vi "Check Action.vi"(6 "HRS Time":dbl, 7 "Values In":dbl[](array[numeric]), 8 "error in (no error)":errorcluster, 11 "Valve in":refnum<class "PeriodicControl.lvclass">) -> (0 "error out":errorcluster, 1 "Do Action":bool, 2 "Action":T1, 3 "Valve out":refnum<class "PeriodicControl.lvclass">, 5 "Values":dbl[](array[numeric]))   [LabVIEW 2020, in "VolatusControl.lvlib" / "PeriodicControl.lvclass"]
uses:
  PeriodicControl.lvclass
  Valve Action.ctl
  Volatus/MessageQ/MessageQ.lvclass
  PeriodicControl.lvclass/PeriodicControl.ctl
  State.ctl
  VolatusControl.lvlib
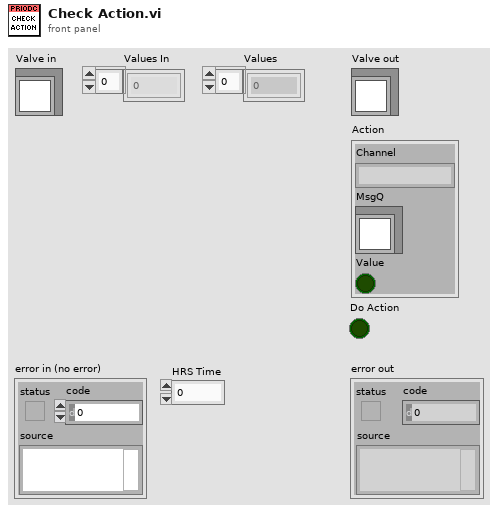
[diagram p1: front panel]
types:
  T1 = typedef "VolatusControl.lvlib/Valve Action.ctl" = cluster{"Channel":string, "MsgQ":refnum<class "MessageQ.lvclass">, "Value":bool}
  T2 = typedef "VolatusControl.lvlib/PeriodicControl.lvclass/State.ctl" = enum16{"Idle", "Start", "Run", "Stop"}
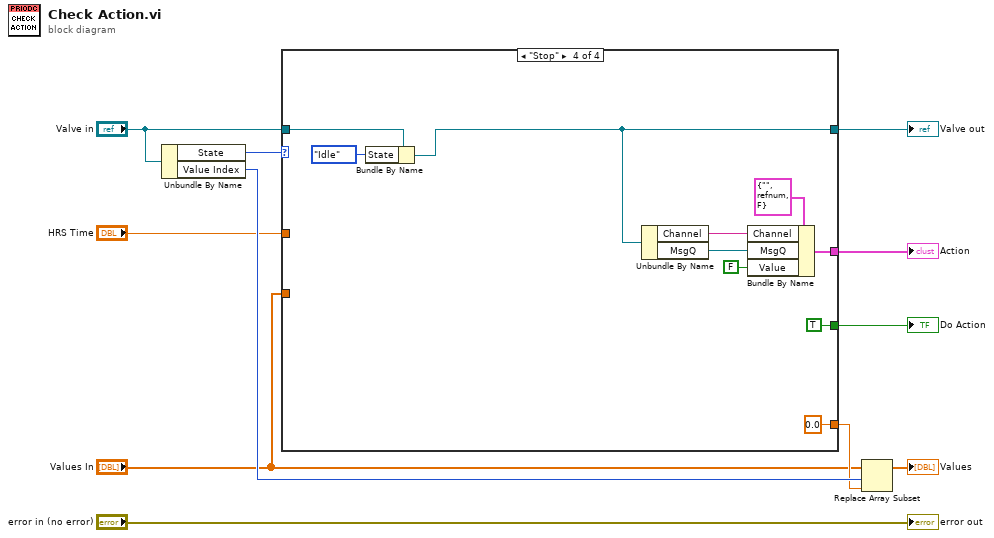
[diagram p0: block diagram]
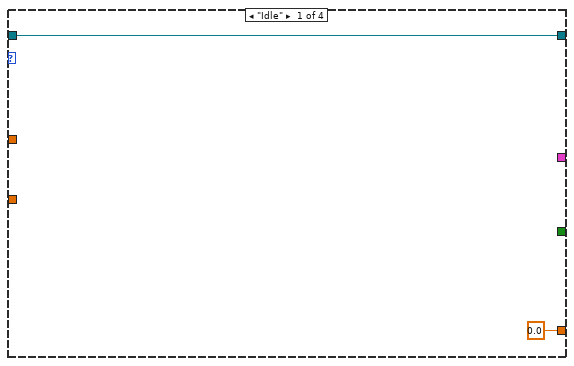
[diagram p2: hidden frame]
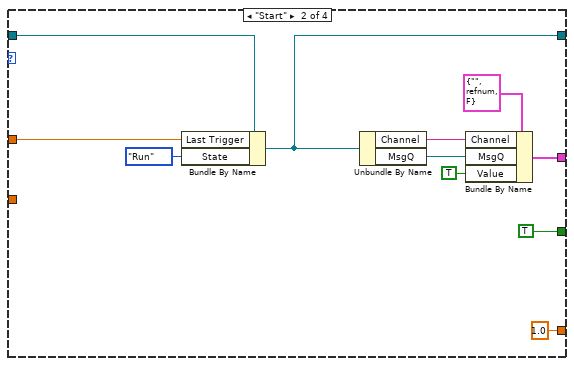
[diagram p3: hidden frame]
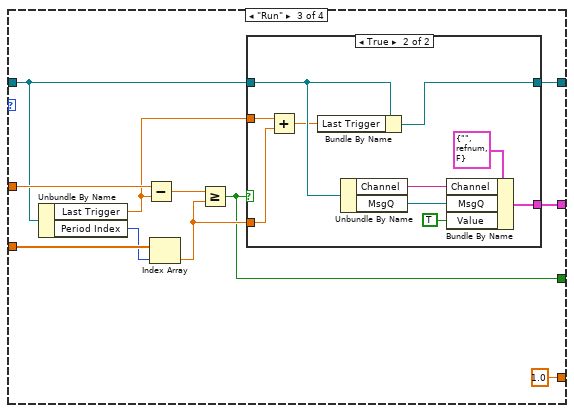
[diagram p4: hidden frame]
diagram:
  n1 = Unbundle By Name("Valve in") -> ("State"=w7:T2, "Value Index"=w9:i32)
  n2 = case shown="\"Stop\"" w7 {
    tunnel: "Valve in" -> [w13 w18 w29 w50]
    tunnel: [w13 w17 w34 w48] -> w6
    tunnel: [0.0 1.0 1.0 0.0] -> w5
    tunnel: "HRS Time" -> [_ w16 w31 _]
    tunnel: [_ TRUE w25 TRUE] -> w3
    tunnel: [_ w22 w35 w51] -> w2
    tunnel: "Values In" -> [_ _ w33 _]
    frame "Idle" {
    }
    frame "Start" {
      n3 = Bundle By Name(cluster=w18, "Last Trigger"=w16, "State"=State."Run") -> (w17:refnum<class "PeriodicControl.lvclass">)
      n4 = Unbundle By Name(w17) -> ("Channel"=w20:string, "MsgQ"=w21:refnum<class "MessageQ.lvclass">)
      n5 = Bundle By Name(cluster=T1 {"Channel"="", "MsgQ"=refnum, "Value"=FALSE} ("Action"), "Channel"=w20, "MsgQ"=w21, "Value"=TRUE) -> (w22:T1)
    }
    frame "Run" {
      n6 = Unbundle By Name(w29) -> ("Last Trigger"=w26:dbl, "Period Index"=w32:i32)
      n7 = Subtract(x=w31, y=w26) -> (x-y=w30:dbl)
      n8 = Index Array(array=w33, index=w32) -> (element=w27:dbl)
      n9 = Greater Or Equal?(x=w30, y=w27) -> (x >= y?=w25:bool)
      n10 = case shown="True" w25 {
        tunnel: [_ w45] -> w35
        tunnel: w29 -> [w36 w40]
        tunnel: [w36 w41] -> w34
        tunnel: w27 -> [_ w38]
        tunnel: w26 -> [_ w39]
        frame False {
        }
        frame True {
          n11 = Add(x=w39, y=w38) -> (x+y=w37:dbl)
          n12 = Bundle By Name(cluster=w40, "Last Trigger"=w37) -> (w41:refnum<class "PeriodicControl.lvclass">)
          n13 = Unbundle By Name(w40) -> ("Channel"=w43:string, "MsgQ"=w44:refnum<class "MessageQ.lvclass">)
          n14 = Bundle By Name(cluster=T1 {"Channel"="", "MsgQ"=refnum, "Value"=FALSE} ("Action"), "Channel"=w43, "MsgQ"=w44, "Value"=TRUE) -> (w45:T1)
        }
      }
    }
    frame "Stop" {
      n15 = Bundle By Name(cluster=w50, "State"=State."Idle") -> (w48:refnum<class "PeriodicControl.lvclass">)
      n16 = Unbundle By Name(w48) -> ("Channel"=w53:string, "MsgQ"=w54:refnum<class "MessageQ.lvclass">)
      n17 = Bundle By Name(cluster=T1 {"Channel"="", "MsgQ"=refnum, "Value"=FALSE} ("Action"), "Channel"=w53, "MsgQ"=w54, "Value"=FALSE) -> (w51:T1)
    }
  }
  "Valve out" <- w6
  "Action" <- w2
  "Do Action" <- w3
  n18 = Replace Array Subset(array="Values In", new element=w5, index=w9) -> (→"Values":dbl[])
  "error out" <- "error in (no error)"
